vi "Get Rx Channel Array.vi"() -> (1 "Channel Array":string[](array[string]))   [LabVIEW 2020, in "AIM ARINC 664 GUID Utility.lvlib"]
uses:
  AIM ARINC 664 GUID Utility.lvlib
  Scripting/Constants.vi
  Scripting/AIM ARINC 664 Scripting.lvlib
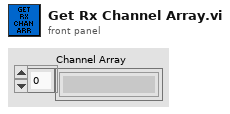
[diagram p1: front panel]
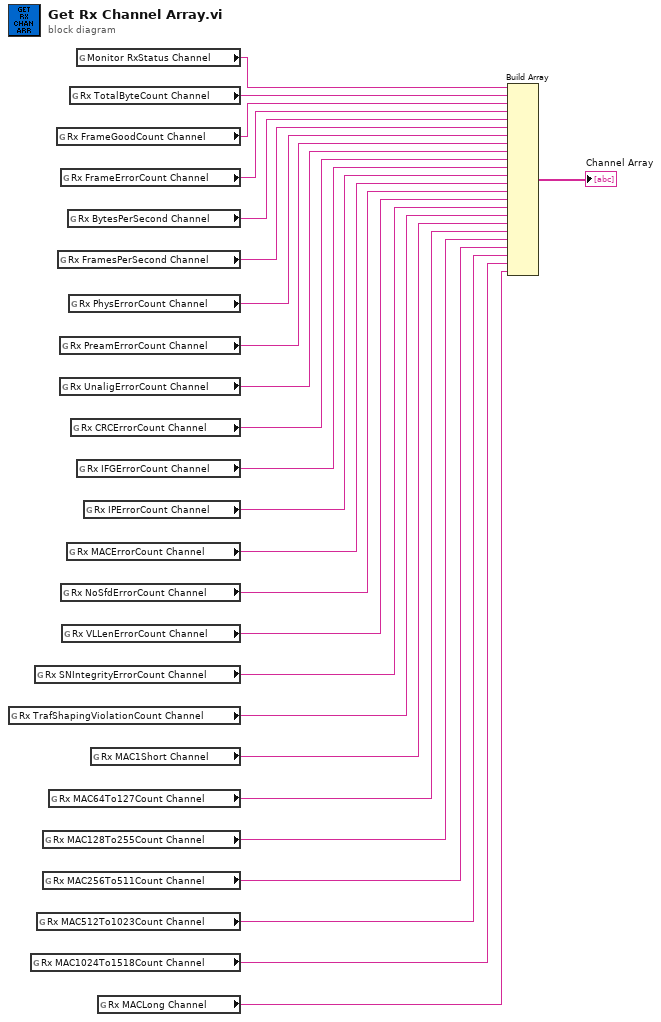
[diagram p0: block diagram]
diagram:
  n1 = global read "Constants.vi" "Rx TrafShapingViolationCount Channel"() -> (w10:string)
  n2 = global read "Constants.vi" "Rx MAC1024To1518Count Channel"() -> (w4:string)
  n3 = global read "Constants.vi" "Rx SNIntegrityErrorCount Channel"() -> (w11:string)
  n4 = global read "Constants.vi" "Rx MAC512To1023Count Channel"() -> (w5:string)
  n5 = global read "Constants.vi" "Rx MAC128To255Count Channel"() -> (w7:string)
  n6 = global read "Constants.vi" "Rx MAC256To511Count Channel"() -> (w6:string)
  n7 = global read "Constants.vi" "Rx MAC64To127Count Channel"() -> (w8:string)
  n8 = global read "Constants.vi" "Rx FrameGoodCount Channel"() -> (w24:string)
  n9 = global read "Constants.vi" "Rx FramesPerSecond Channel"() -> (w21:string)
  n10 = global read "Constants.vi" "Rx PreamErrorCount Channel"() -> (w19:string)
  n11 = global read "Constants.vi" "Rx UnaligErrorCount Channel"() -> (w18:string)
  n12 = global read "Constants.vi" "Rx FrameErrorCount Channel"() -> (w23:string)
  n13 = global read "Constants.vi" "Rx NoSfdErrorCount Channel"() -> (w13:string)
  n14 = global read "Constants.vi" "Rx VLLenErrorCount Channel"() -> (w12:string)
  n15 = global read "Constants.vi" "Rx MACErrorCount Channel"() -> (w14:string)
  n16 = global read "Constants.vi" "Rx BytesPerSecond Channel"() -> (w22:string)
  n17 = global read "Constants.vi" "Rx PhysErrorCount Channel"() -> (w20:string)
  n18 = global read "Constants.vi" "Rx TotalByteCount Channel"() -> (w25:string)
  n19 = global read "Constants.vi" "Rx CRCErrorCount Channel"() -> (w17:string)
  n20 = global read "Constants.vi" "Monitor RxStatus Channel"() -> (w1:string)
  n21 = global read "Constants.vi" "Rx IFGErrorCount Channel"() -> (w16:string)
  n22 = global read "Constants.vi" "Rx IPErrorCount Channel"() -> (w15:string)
  n23 = global read "Constants.vi" "Rx MAC1Short Channel"() -> (w9:string)
  n24 = global read "Constants.vi" "Rx MACLong Channel"() -> (w3:string)
  n25 = Build Array(w1, w25, w24, w23, w22, w21, w20, w19, w18, w17, w16, w15, w14, w13, w12, w11, w10, w9, w8, w7, w6, w5, w4, w3) -> (→"Channel Array":string[])
